vi "2阶系统仿真.vi"() -> ()   [LabVIEW 2014]
uses:
  <vilib>/addons/Control Design/_Model Construction/Special Model Creation.llb/Special Model Creation SubVI/CD Create 2nd Order Model.vi
  <vilib>/addons/Control Design/_Time Response Analysis/Time Response.llb/Time Response subVI/cd_Step Response (Transfer Function).vi
  <vilib>/addons/Control Design/_Time Response Analysis/Time Response.llb/Time Response subVI/cd_Impulse Response (Transfer Function).vi
  <vilib>/addons/Control Design/_Time Response Analysis/Time Response.llb/Time Response subVI/cd_Parametric Time Response (TF).vi
  <vilib>/addons/Control Design/_Utility/Model Viewer.llb/Model Viewer SubVI/cd_Draw Transfer Function Equation (TF).vi
  <vilib>/addons/Control Design/_Model Construction/NI_CD_Special Model Creation.lvlib
  <vilib>/addons/Control Design/_Utility/NI_CD_Model Viewer.lvlib
  <vilib>/addons/Control Design/_Time Response Analysis/NI_CD_Time Response.lvlib
panel:
  out "峰值":dbl[][](array[numeric])
  out "稳态裕量":dbl[][](array[numeric])
  out "超调量 (%)":dbl[][](array[numeric])
  out "调整时间 (s)":dbl[][](array[numeric])
  out "高峰时间 (s)":dbl[][](array[numeric])
  out "上升时间 (s)":dbl[][](array[numeric])
  out "Time Response":cluster{"time":dbl[], dbl[]}[](graph) caption="时间特性图"
  out "阶跃特性图":cluster{"time":dbl[], dbl[]}[](graph)
  out "脉冲特性图":cluster{"time":dbl[], dbl[]}[](graph) caption="Impulse Response Graph"
  out "Resulting Model 2":picture
  in  "z":dbl(knob)=0.5 scale=0.0..2.0
  in  "wn":dbl(knob)=4.0 scale=0.1..3.0
  in  "Gain (K)":dbl(slide)=1.0 scale=-8.0..8.0
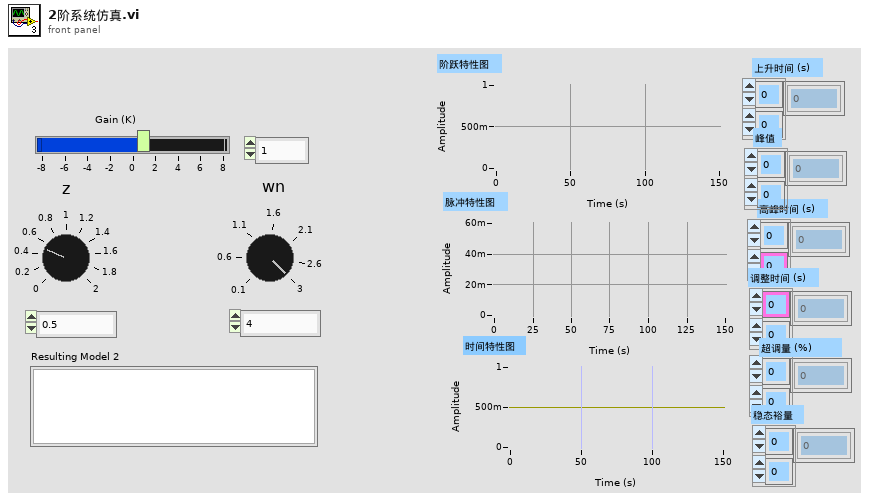
[diagram p1: front panel]
types:
  T1 = typedef "NI_LinSys_Model Typedefs.lvlib/CD Transfer Function Model (MIMO).ctl" = cluster{"properties":T2, "transfer function(s)":T3[][]}
  T2 = typedef "NI_LinSys_Model Typedefs.lvlib/CD General Elements.ctl" = cluster{"Model name":string, "Input names":string[], "Output names":string[], "Input Delays":dbl[], "Output Delays":dbl[], "Sampling Time":dbl, "Notes":string}
  T3 = typedef "NI_LinSys_Model Typedefs.lvlib/CD Transfer Function Model (SISO).ctl" = cluster{"Numerator":dbl[], "Denominator":dbl[], "delay":dbl}
  T4 = typedef "NI_LinSys_Data Typedefs.lvlib/CD Parametric Time Response Data.ctl" = cluster{"Rise Time (s)":dbl[][], "Peak Time (s)":dbl[][], "Settling Time (s)":dbl[][], "Overshoot (%)":dbl[][], "Steady-State Gain":dbl[][], "Peak Value":dbl[][]}
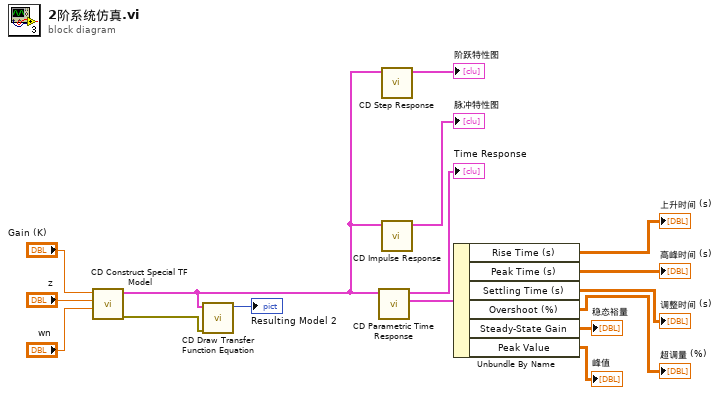
[diagram p0: block diagram]
diagram:
  n1 = call-poly <vilib>:"CD Construct Special TF Model.vi"("Natural Frequency (rad/s)"="wn", "Damping Ratio"="z", "Static Gain"="Gain (K)") -> ("error out"=w5:errorcluster, "Transfer Function Model"=w1:T1)  [unwired: 7 in]
  n2 = call-poly <vilib>:"CD Draw Transfer Function Equation.vi"("error in (no error)"=w5, "Transfer Function Model"=w1) -> ("Equation"=→"Resulting Model 2":picture)  [unwired: 7 in, 2 out]
  n3 = call-poly <vilib>:"CD Parametric Time Response.vi"("Transfer Function Model"=w1) -> ("Time Response Parametric Data"=w13:T4, "Time Response"=→"Time Response":cluster{"time":dbl[], dbl[]}[])  [unwired: 7 in, 2 out]
  n4 = call-poly <vilib>:"CD Step Response.vi"("Transfer Function Model"=w1) -> ("Step Response Graph"=→"阶跃特性图":cluster{"time":dbl[], dbl[]}[])  [unwired: 8 in, 2 out]
  n5 = call-poly <vilib>:"CD Impulse Response.vi"("Transfer Function Model"=w1) -> ("Impulse Response Graph"=→"脉冲特性图":cluster{"time":dbl[], dbl[]}[])  [unwired: 8 in, 2 out]
  n6 = Unbundle By Name(w13) -> ("Rise Time (s)"=→"上升时间 (s)":dbl[][], "Peak Time (s)"=→"高峰时间 (s)":dbl[][], "Settling Time (s)"=→"调整时间 (s)":dbl[][], "Overshoot (%)"=→"超调量 (%)":dbl[][], "Steady-State Gain"=→"稳态裕量":dbl[][], "Peak Value"=→"峰值":dbl[][])
